vi "Acceleration.vi"() -> ()   [LabVIEW 2020]
uses:
  Control/AccelerationBestRecordIndicator.ctl
  Control/AccelerationCurrentRecordIndicator.ctl
  CommonControl/Flag.ctl
  Control/AccelerationState.ctl
  <vilib>/DAQmx/write.llb/DAQmx Write (Analog 1D DBL NChan 1Samp).vi
  <vilib>/DAQmx/read.llb/DAQmx Read (Analog 1D DBL NChan 1Samp).vi
  <vilib>/DAQmx/create/channels.llb/DAQmx Create Channel (AO-Voltage-Basic).vi
  <vilib>/DAQmx/create/channels.llb/DAQmx Create Channel (AI-Voltage-Basic).vi
  <vilib>/Utility/file.llb/Read Delimited Spreadsheet (string).vi
  <vilib>/DAQmx/miscellaneous.llb/DAQmx Fill In Error Info.vi
  <vilib>/Utility/file.llb/Write Delimited Spreadsheet (string).vi
panel:
  in  "DNF":bool
  out "Event ProgressData":string[][](table)
  in  "DAQDevice":tag
  in  "NextEntry":bool
  in  "Ready":bool
  in  "Retry":bool
  out "CurrentRecordIndicator":T1
  out "BestRecordIndicator":T2
  in  "Stop":bool
  # "2022 KSAE Formula Acceleration Event"
  # "Time :"
  # "Entry :"
  # "#1"
  # "#2"
  # "#3"
  # "#4"
  # "Univ. :"
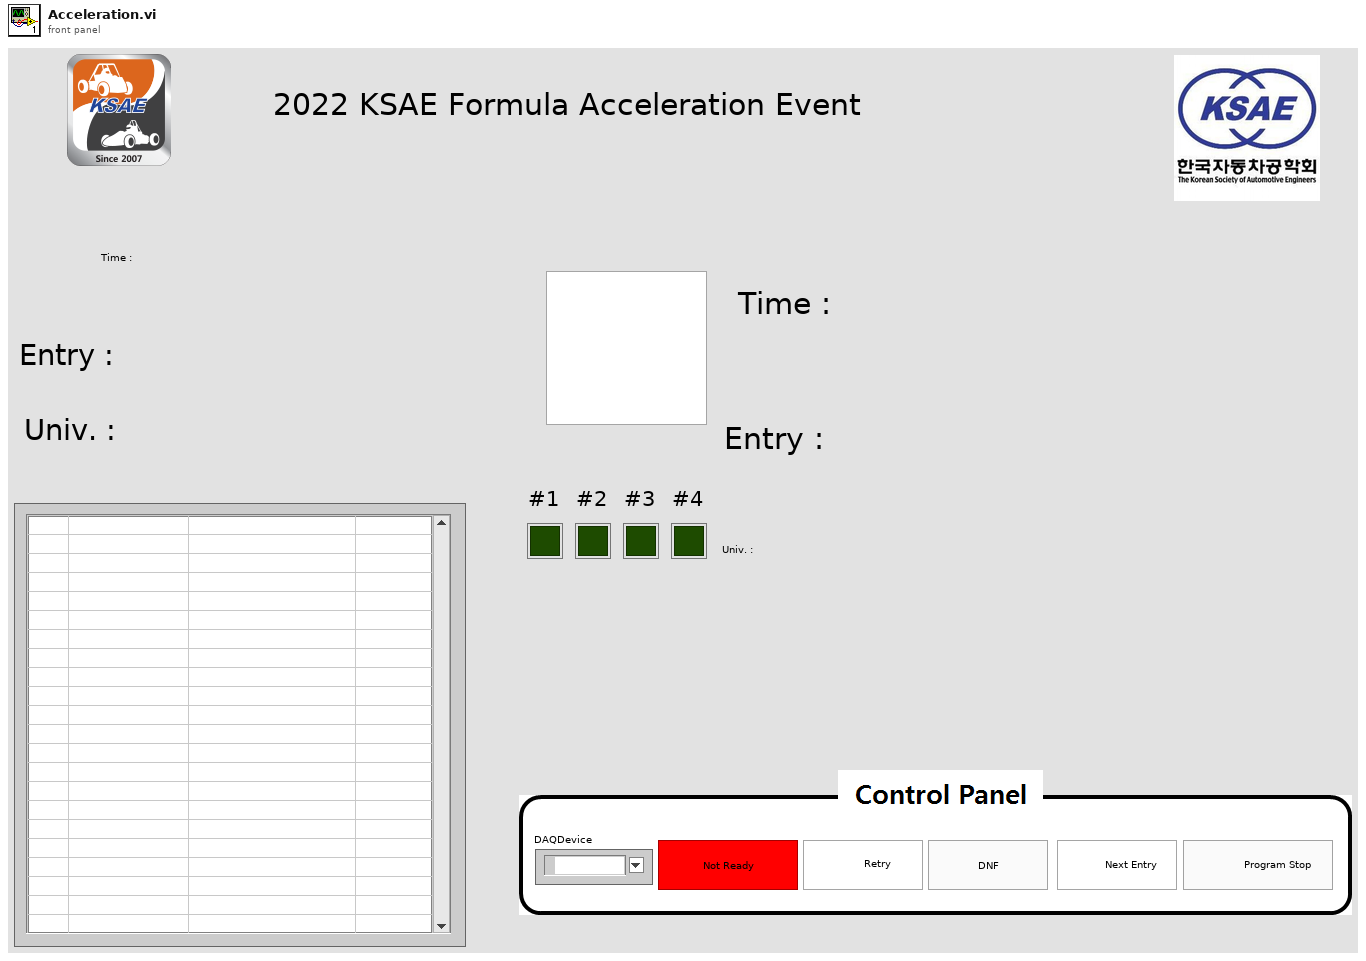
[diagram p1: front panel]
types:
  T1 = typedef "AccelerationCurrentRecordIndicator.ctl" = cluster{"Flag":picture, "Message":string, "Attempt":cluster{"Attempt-1":bool, "Attempt-2":bool, "Attempt-3":bool, "Attempt-4":bool}, "CurrentTime":string, "CurrentEntry":string, "CurrentUniversity":string}
  T2 = typedef "AccelerationBestRecordIndicator.ctl" = cluster{"BestTime":string, "BestEntry":string, "BestUniv":string}
  T3 = typedef "Flag.ctl" = cluster{"GreenFlag":picture, "BlueFlag":picture, "RedFlag":picture, "CheckFlag":picture}
  T4 = typedef "AccelerationState.ctl" = enum16{"Initial", "InputInfomation", "Ready", "Running", "FinshRunning", "LogRecord", "HardwareRelease", "WaittingforNext", "ProgramStop"}
  T5 = cluster{"CurrentRecordIndicator":T1, "BestRecordIndicator":T2, "FlageData":T3, "RefTime(msec)":i64, "Time(msec)":i64, "StateValue":T4, "EventProgress":sgl, "EventProgressData":string[][], "Ready":bool, "Retry":bool, "DNF":bool, "NextEntry":bool, "Stop":bool}
  T6 = cluster{"CurrentEntry":string, "CurrentUniversity":string, "CurrentTeam":string}
  T7 = cluster{"Attempt-1":bool, "Attempt-2":bool, "Attempt-3":bool, "Attempt-4":bool}
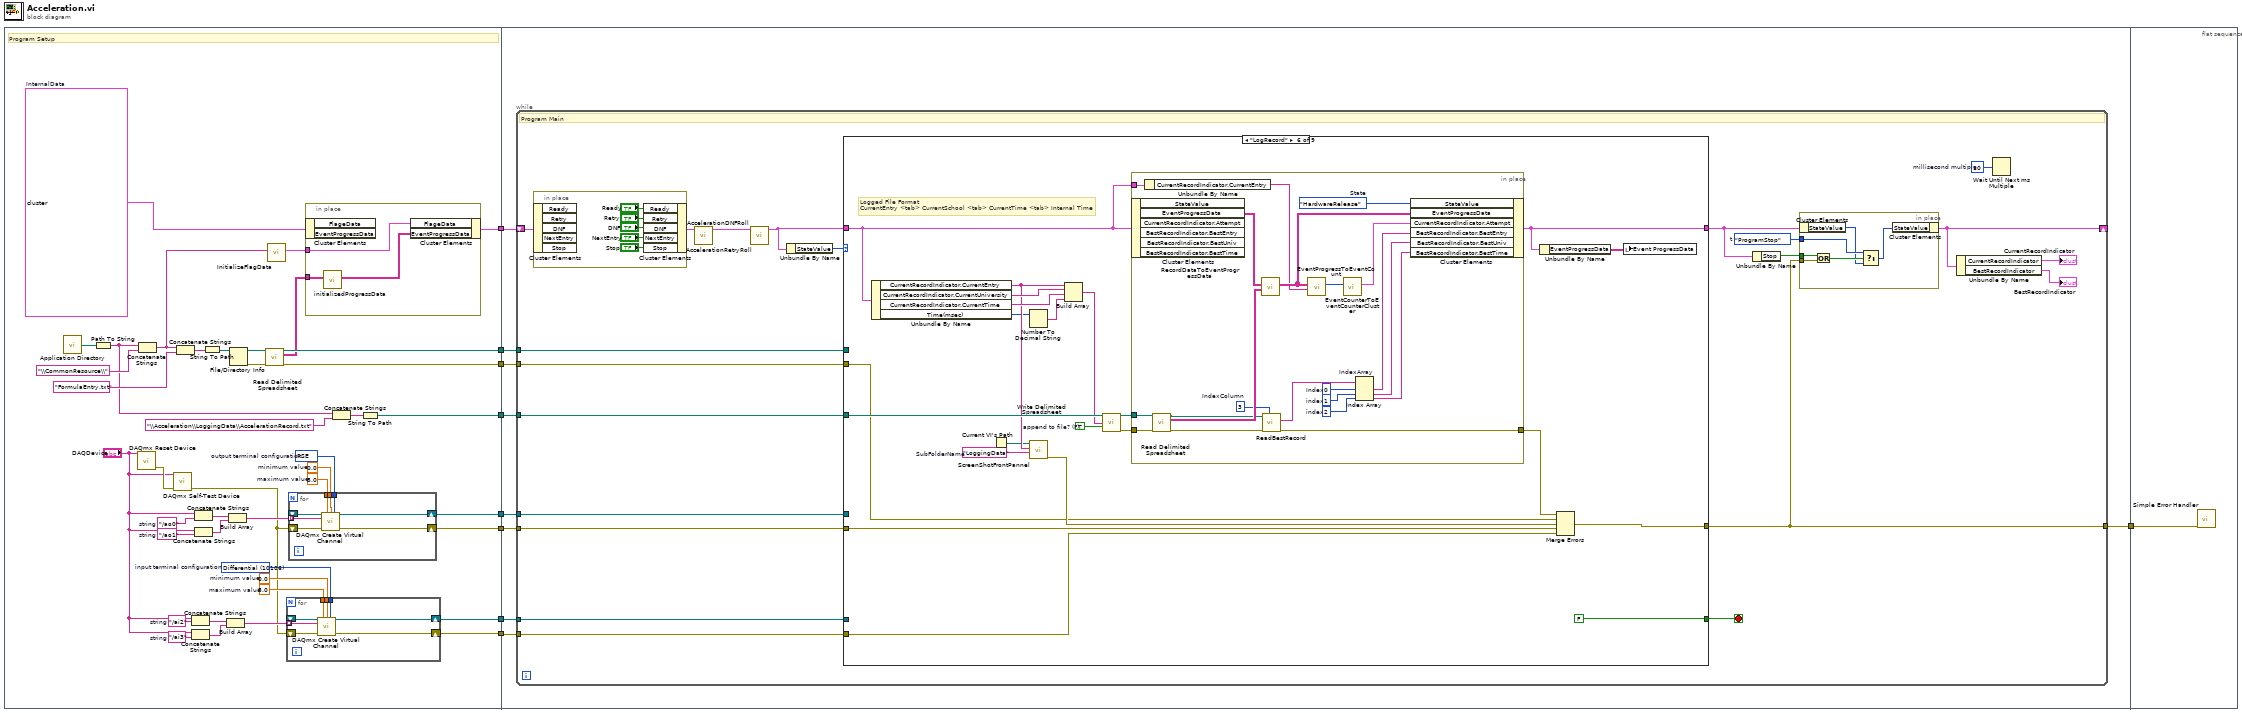
[diagram p0: block diagram]
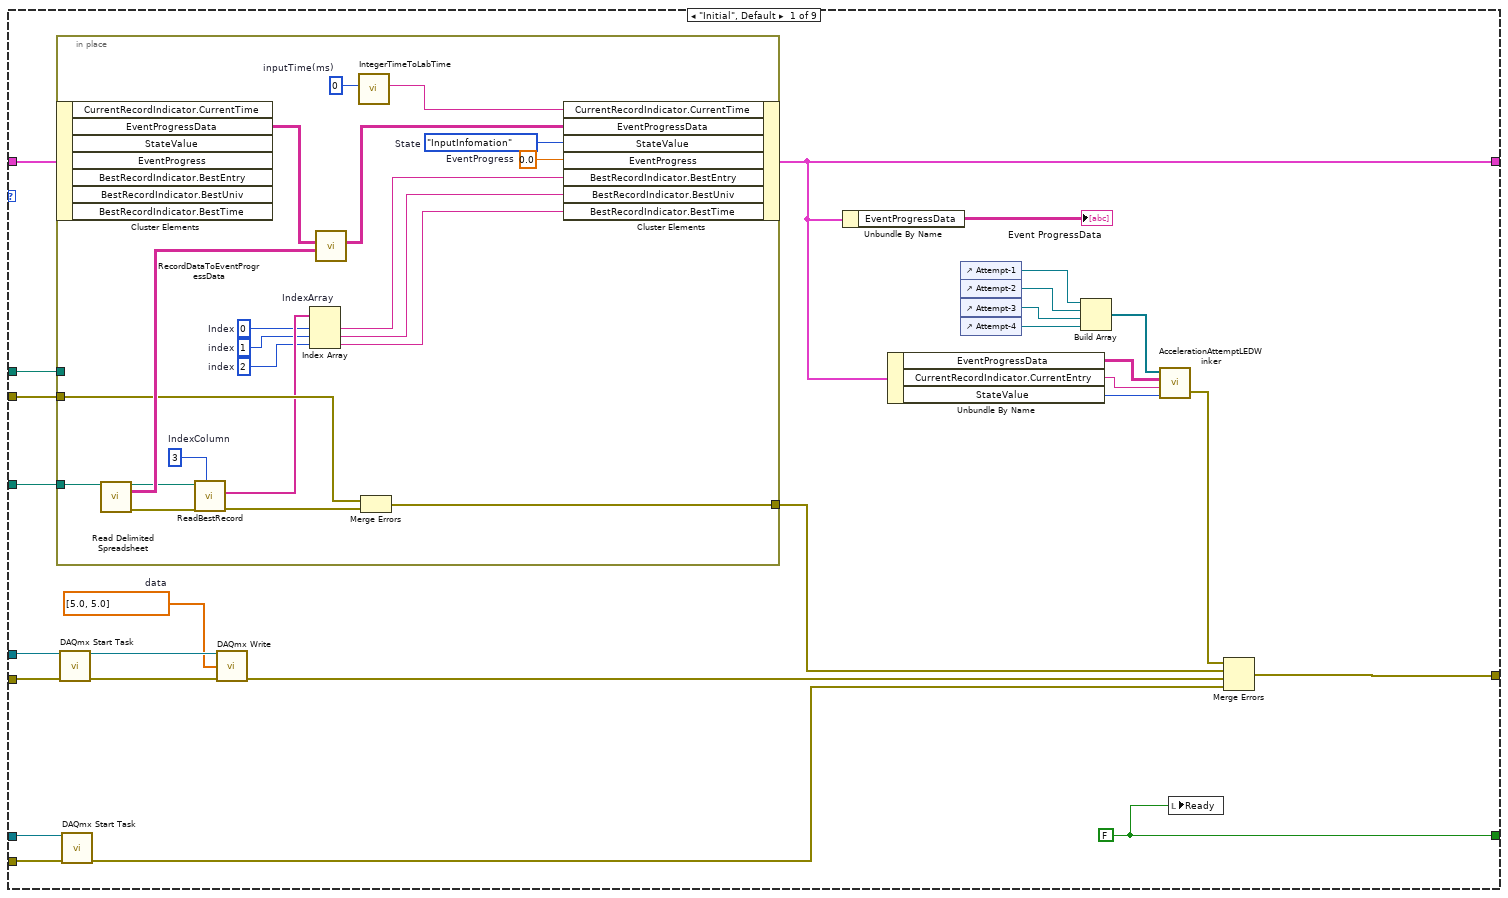
[diagram p2: hidden frame]
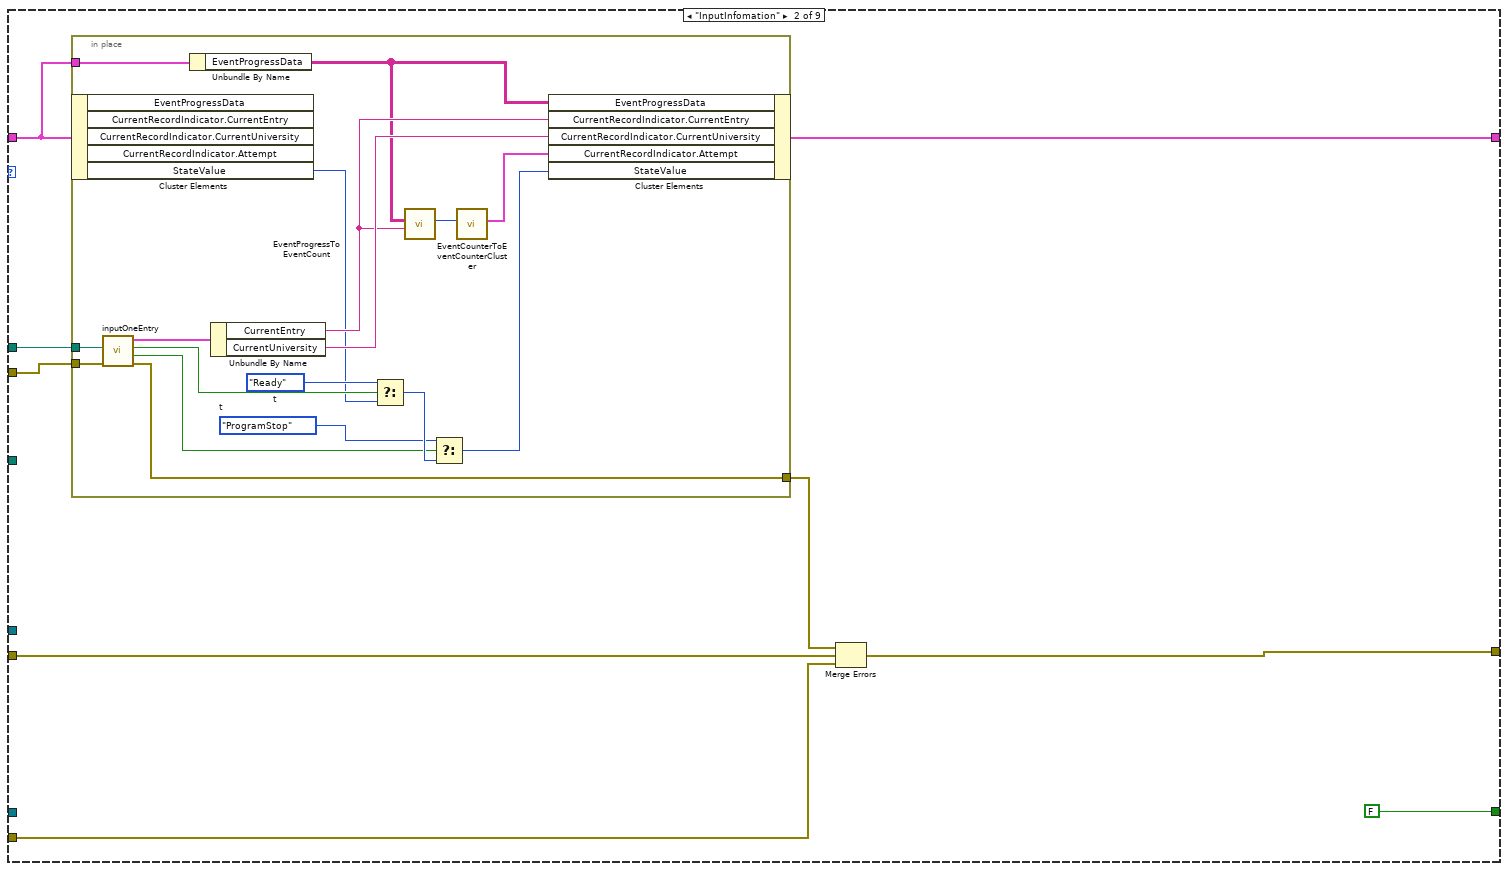
[diagram p3: hidden frame]
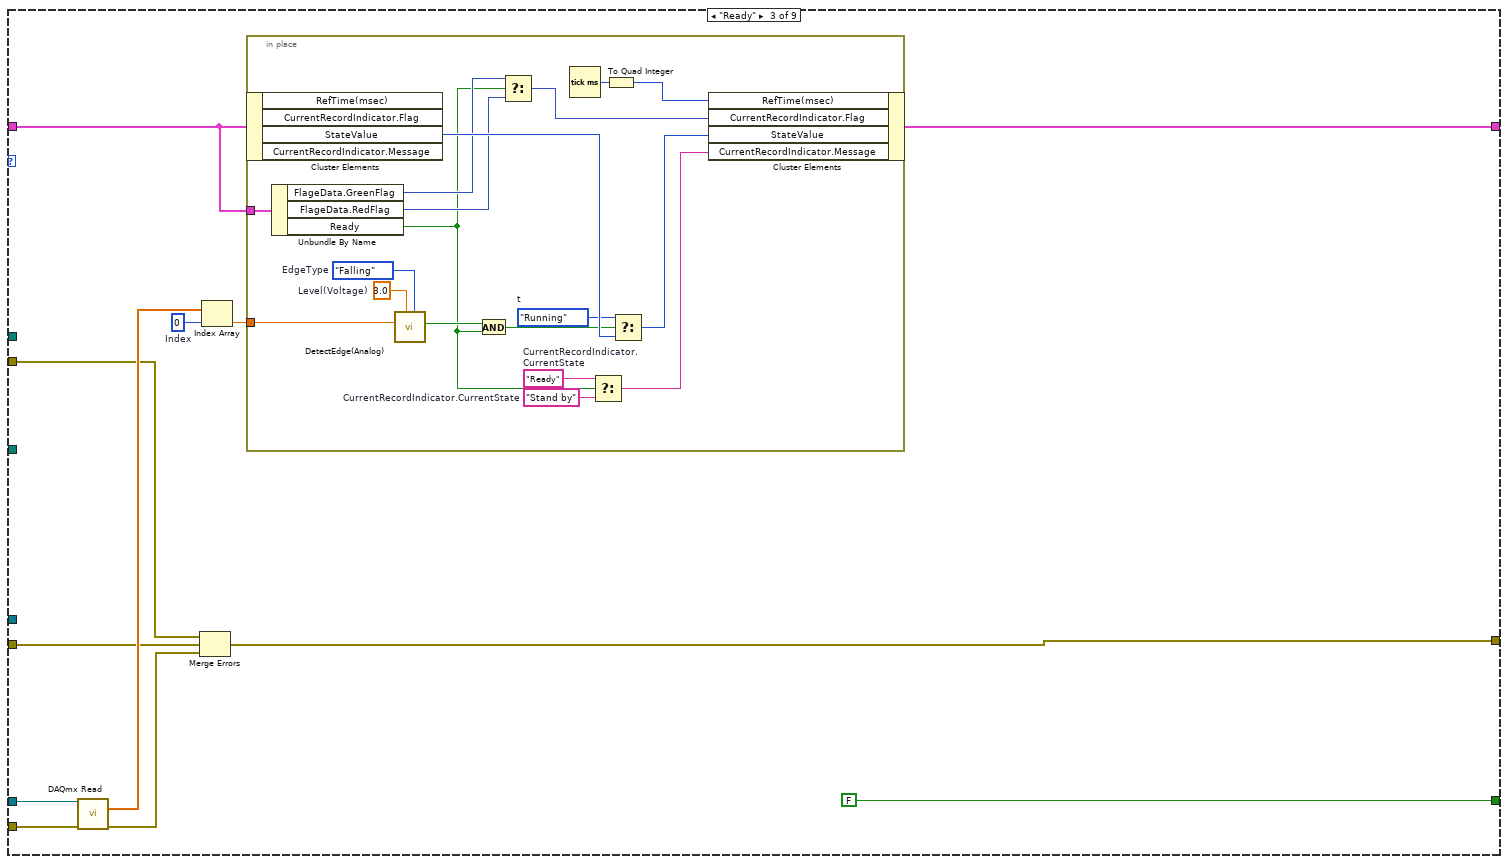
[diagram p4: hidden frame]
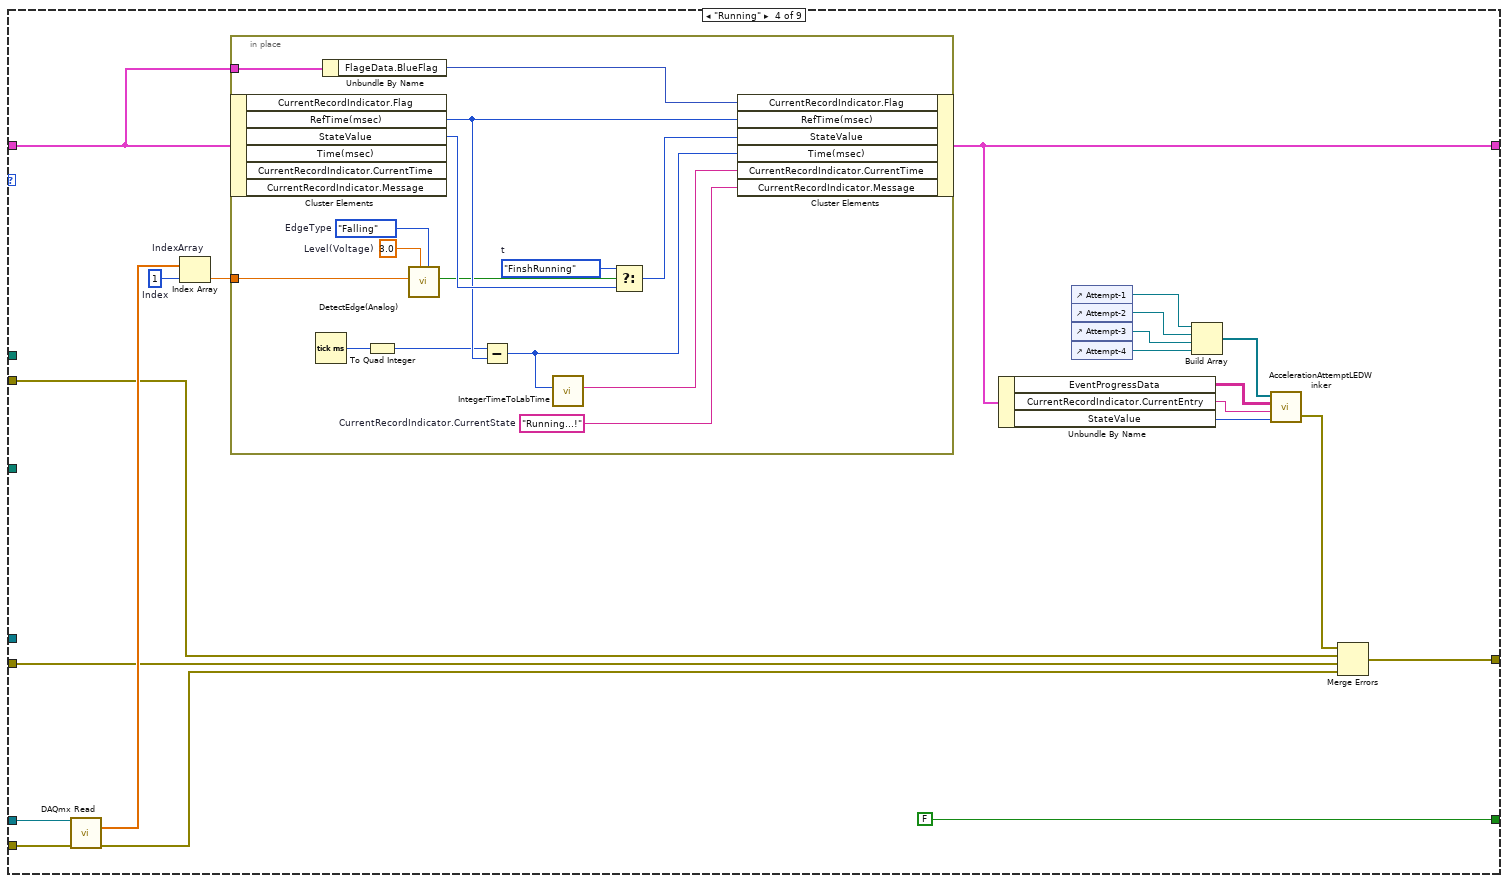
[diagram p5: hidden frame]
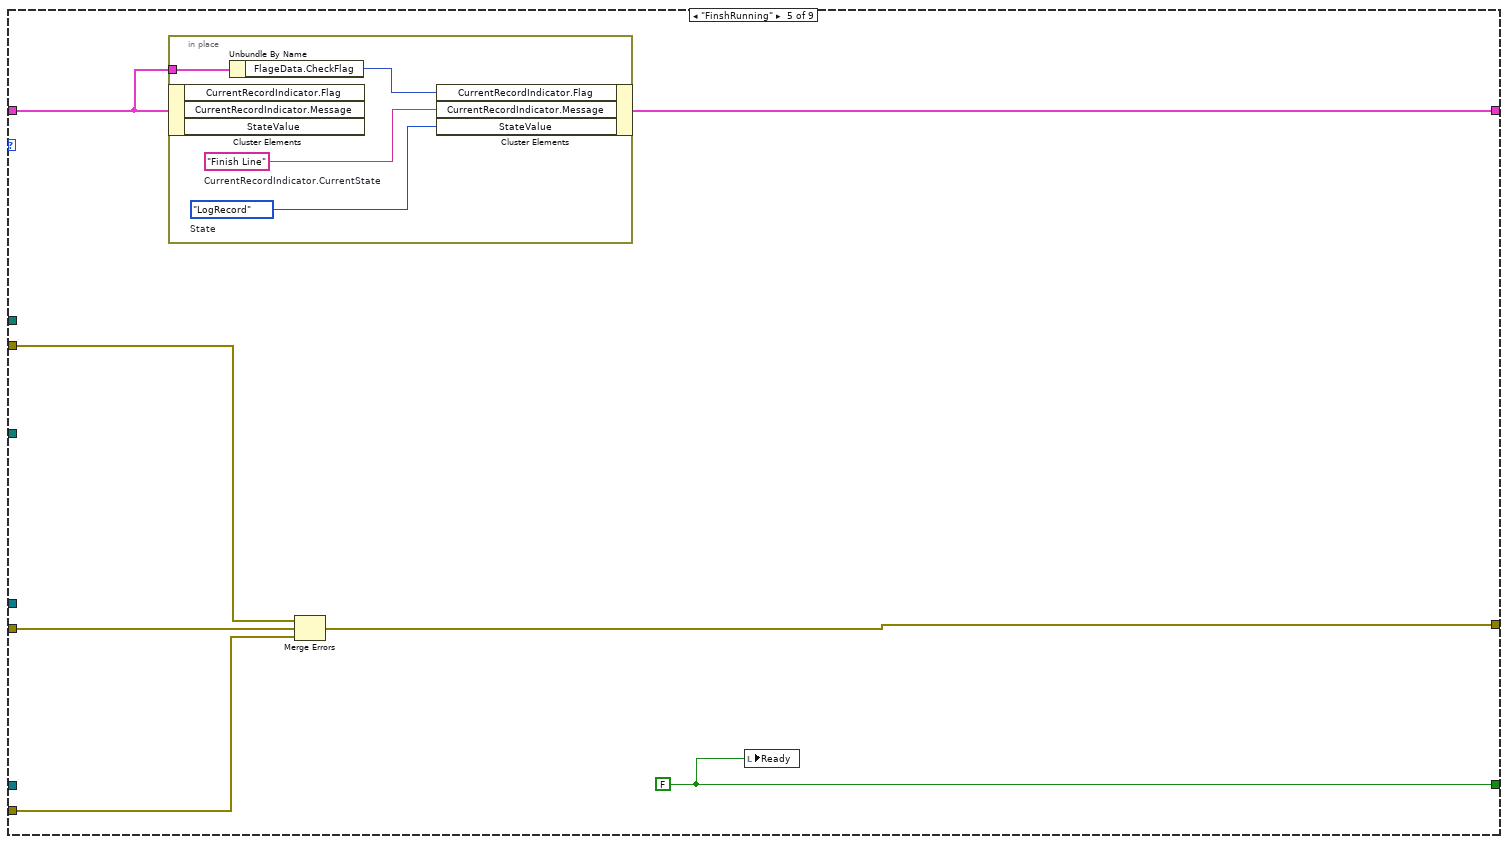
[diagram p6: hidden frame]
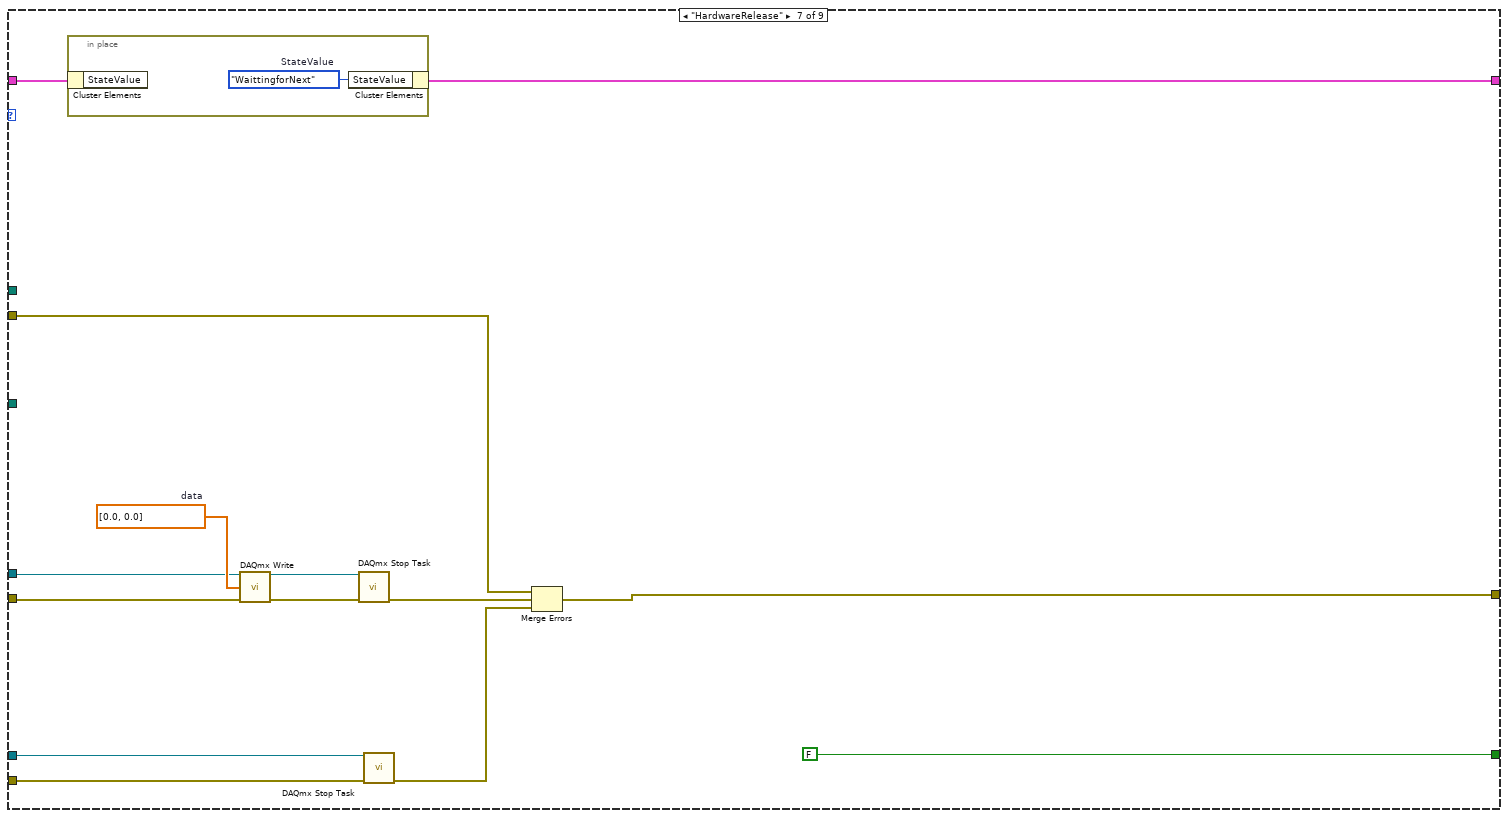
[diagram p7: hidden frame]
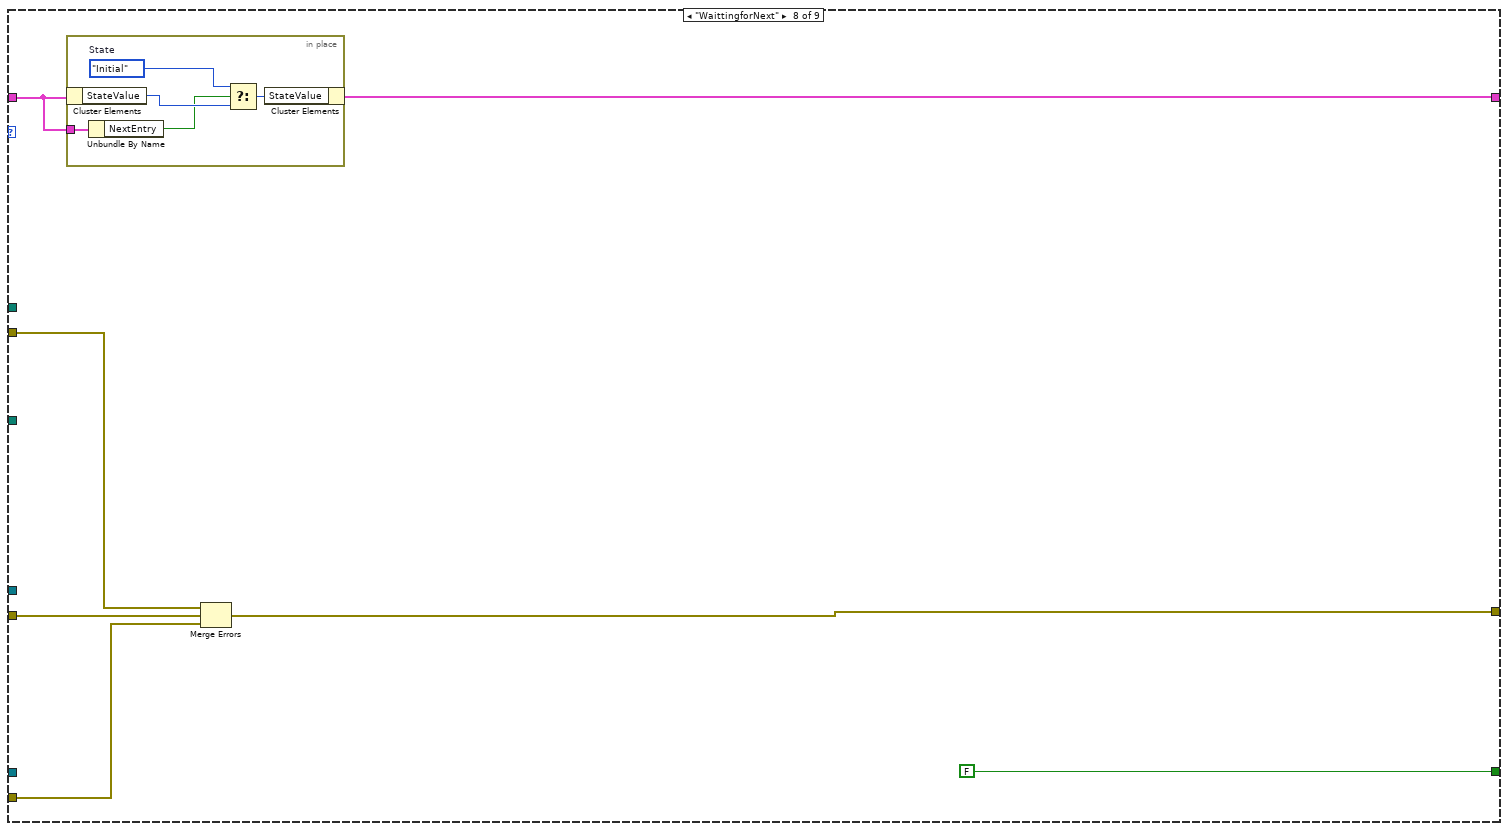
[diagram p8: hidden frame]
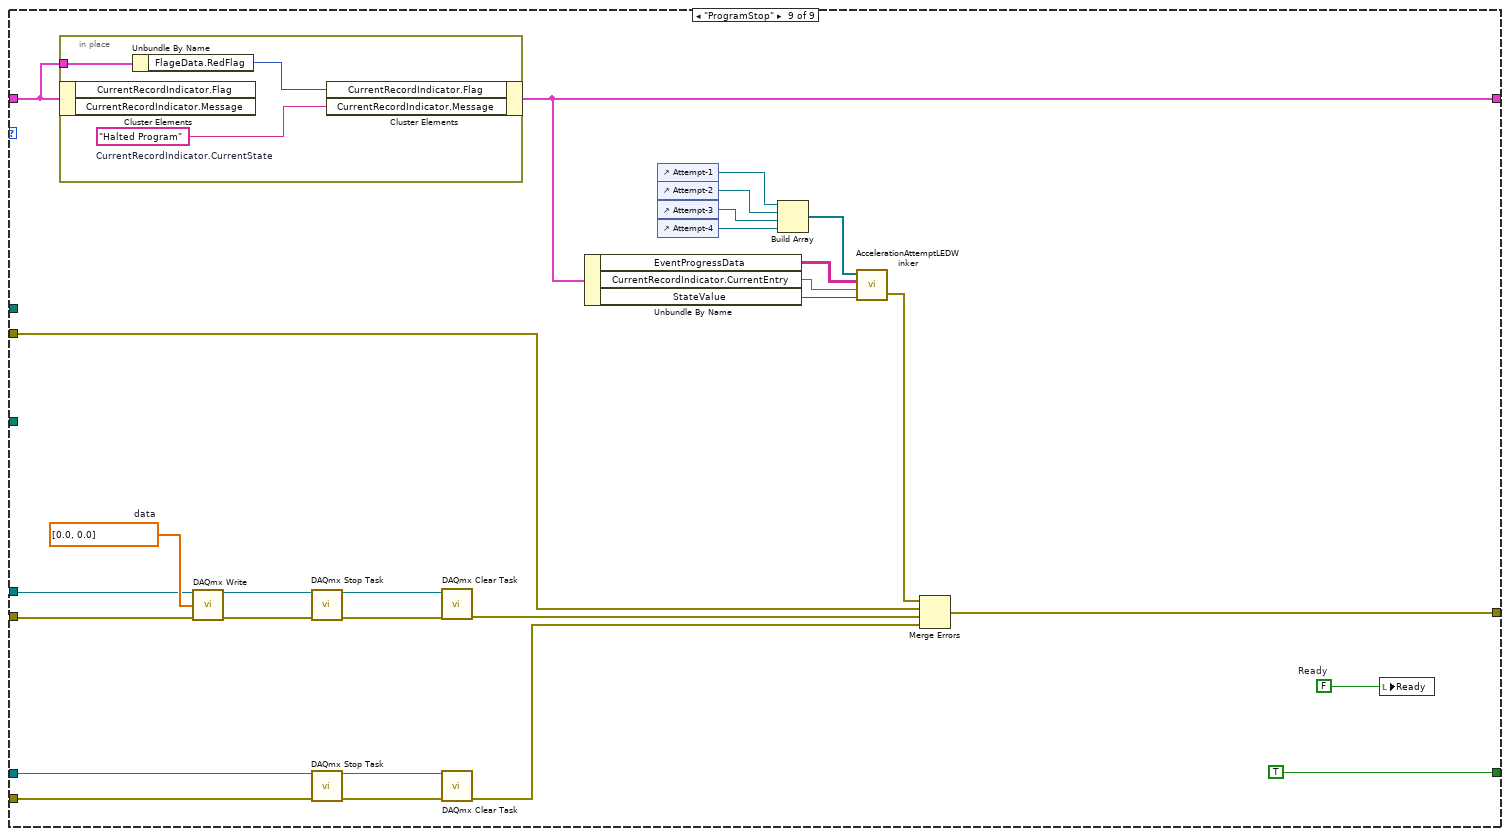
[diagram p9: hidden frame]
diagram:
  n1 = flat-sequence {
    tunnel: [w49] -> w9
    tunnel: [w47] -> w8
    tunnel: [w35] -> w7
    tunnel: [w13] -> w6
    tunnel: [w22] -> w5
    tunnel: [w20] -> w4
    tunnel: [w16] -> w3
    tunnel: [w15] -> w2
    tunnel: w9 -> [w72]
    tunnel: w8 -> [w74]
    tunnel: w7 -> [w75]
    tunnel: w6 -> [w76]
    tunnel: w5 -> [w77]
    tunnel: w4 -> [w69]
    tunnel: w3 -> [w73]
    tunnel: w2 -> [w71]
    tunnel: [w70] -> w1
    tunnel: w1 -> [w362]
    frame #0 {
      w14 = T5 {"CurrentRecordIndicator"={"Flag"=bytes[0], "Message"="", "Attempt"={"Attempt-1"=FALSE, "Attempt-2"=FALSE, "Attempt-3"=FALSE, "Attempt-4"=FALSE}, "CurrentTime"="", "CurrentEntry"="", "CurrentUniversity"=""}, "BestRecordIndicator"={"BestTime"="", "BestEntry"="", "BestUniv"=""}, "FlageData"={"GreenFlag"=bytes[0], "BlueFlag"=bytes[0], "RedFlag"=bytes[0], "CheckFlag"=bytes[0]}, "RefTime(msec)"=0, "Time(msec)"=0, "StateValue"=enum."Initial", "EventProgress"=0.0, "EventProgressData"=[], "Ready"=FALSE, "Retry"=FALSE, "DNF"=FALSE, "NextEntry"=FALSE, "Stop"=FALSE}  # InternalData
      w26 = "/ai3"  # string
      w27 = "/ai2"  # string
      w29 = "/ao1"  # string
      w31 = "/ao0"  # string
      w33 = 5.0  # maximum value
      w32 = 0.0  # minimum value
      w34 = 10106 items=["default"=-1, "RSE"=10083, "NRSE"=10078, "Differential"=10106, "Pseudodifferential"=12529]  # input terminal configuration
      w43 = 10083 items=["Default"=-1, "RSE"=10083, "Differential"=10106, "Pseudodifferential"=12529]  # output terminal configuration
      w44 = 0.0  # minimum value
      w45 = 5.0  # maximum value
      # "Program Setup"
      n2 = call <vilib>:"Application Directory.vi"() -> ("Application Directory"=w42:path)
      n3 = Path To String(path=w42) -> (string=w37:string)
      n4 = call <vilib>:"DAQmx Reset Device.vi"("device in"="DAQDevice") -> ("error out"=w19:errorcluster)  [unwired: 14 in]
      n5 = Concatenate Strings "Concatenate Strings"(w37, "\\CommonResource\\") -> (w11:string)
      n6 = call <vilib>:"DAQmx Self-Test Device.vi"("device in"="DAQDevice", "error in"=w19) -> ("error out"=w17:errorcluster)  [unwired: 13 in]
      n7 = Concatenate Strings(w11, "FormulaEntry.txt") -> (w36:string)
      n8 = Concatenate Strings "Concatenate Strings"("DAQDevice", w27) -> (w25:string)
      n9 = Concatenate Strings "Concatenate Strings"("DAQDevice", w26) -> (w24:string)
      n10 = Concatenate Strings "Concatenate Strings"("DAQDevice", w31) -> (w30:string)
      n11 = Concatenate Strings "Concatenate Strings"("DAQDevice", w29) -> (w28:string)
      n12 = String To Path(string=w36) -> (path=w23:path)
      n13 = Build Array "Build Array"(w25, w24) -> (w48:string[])
      n14 = Build Array "Build Array"(w30, w28) -> (w46:string[])
      n15 = File/Directory Info(path=w23) -> (path out=w22:path, error out=w21:errorcluster)  [unwired: 1 in, 5 out]
      n16 = call-poly <vilib>:"Read Delimited Spreadsheet.vi"("file path (dialog if empty)"=w22, "error in (no error)"=w21) -> ("all rows"=w12:string[][], "error out"=w20:errorcluster)  [unwired: 8 in, 4 out]
      n17 = call "InitializeFlagData.vi"("inputPath"=w11) -> ("outputFlagData"=w10:T3)  [unwired: 9 in, 1 out]
      n18 = for {
        tunnel: w34 -> [w68]
        shift-right: [w67] -> w15
        shift-left: w17 -> [w64]
        shift-right: [w66] -> w49
        shift-left: _ -> [w65]
        tunnel: w33 -> [w63]
        tunnel: w32 -> [w62]
        tunnel: w48 -> [w61] mode=indexing
        n19 = call-poly <vilib>:"DAQmx Create Virtual Channel.vi"("task in"=w65, "maximum value"=w63, "minimum value"=w62, "input terminal configuration"=w68, "physical channels"=w61, "error in"=w64) -> ("task out"=w66:refnum<k21>, "error out"=w67:errorcluster)  [unwired: 8 in]
      }
      n20 = for {
        shift-right: [w60] -> w47
        shift-left: _ -> [w57]
        shift-right: [w59] -> w16
        shift-left: w17 -> [w56]
        tunnel: w46 -> [w58] mode=indexing
        tunnel: w45 -> [w55]
        tunnel: w44 -> [w54]
        tunnel: w43 -> [w53]
        n21 = call-poly <vilib>:"DAQmx Create Virtual Channel.vi"("task in"=w57, "maximum value"=w55, "minimum value"=w54, "output terminal configuration"=w53, "physical channels"=w58, "error in"=w56) -> ("task out"=w60:refnum<k21>, "error out"=w59:errorcluster)  [unwired: 8 in]
      }
      n22 = in-place {
        in-place-border: w10 -> [w50]
        in-place-border: w12 -> [w52]
        n23 = in-place-cluster #1(w14) -> ()  [unwired: 2 out]
        n24 = call "initializedProgressData.vi"("inputEntry"=w52) -> ("outputProgressData"=w51:string[][])  [unwired: 10 in]
        n25 = in-place-cluster #1("FlageData"=w50, "EventProgressData"=w51) -> (w13:T5)
      }
      n26 = Concatenate Strings "Concatenate Strings"(w37, "\\Acceleration\\LoggingData\\AccelerationRecord.txt") -> (w40:string)
      n27 = String To Path(string=w40) -> (path=w35:path)
    }
    frame #1 {
      n28 = while {
        tunnel: w72 -> [w98]
        shift-right: [w84] -> _
        shift-left: w76 -> [w88]
        tunnel: w74 -> [w94]
        tunnel: w75 -> [w93]
        tunnel: w77 -> [w91]
        tunnel: w73 -> [w90]
        tunnel: w71 -> [w89]
        tunnel: [w78] -> w70
        tunnel: w69 -> [w87]
        stop <- w95 stop-if-true
        w85 = AccelerationState."ProgramStop"  # t
        w92 = u32 10  # millisecond multiple
        # "Program Main"
        n29 = in-place {
          n30 = in-place-cluster #2(w88) -> ()  [unwired: 5 out]
          n31 = in-place-cluster #2("Ready"="Ready", "Retry"="Retry", "DNF"="DNF", "NextEntry"="NextEntry", "Stop"="Stop") -> (w82:T5)
        }
        n32 = call "AccelerationDNFRoll.vi"("inputInternalData"=w82) -> ("outputInternalData"=w81:T5)  [unwired: 10 in]
        n33 = call "AccelerationRetryRoll.vi"("inputInternalData"=w81) -> ("outputInternalData"=w80:T5)  [unwired: 10 in]
        n34 = Unbundle By Name(w80) -> ("StateValue"=w79:T4)
        n35 = case shown="\"LogRecord\"" w79 {
          tunnel: w98 -> [w124 _ w189 w228 _ _ w306 _ w352]
          tunnel: w89 -> [w123 w153 w188 w227 w249 w266 w305 w316 w338]
          tunnel: w80 -> [w130 w152 w181 w221 w248 w257 w300 w313 w336]
          tunnel: [w106 w157 w187 w210 w250 w265 w299 w318 w327] -> w83
          tunnel: [w105 FALSE FALSE FALSE w244 FALSE FALSE FALSE TRUE] -> w95
          tunnel: [w120 w159 w180 w220 w247 w272 w302 w317 w348] -> w78
          tunnel: w94 -> [w126 _ _ _ _ _ w308 _ w343]
          tunnel: w93 -> [w116 _ _ _ _ w273 _ _ _]
          tunnel: w91 -> [w119 w156 _ _ _ _ _ _ _]
          tunnel: w90 -> [w125 w154 w179 w219 w246 w267 w307 w315 w342]
          tunnel: w87 -> [w118 w155 w178 w218 w245 w256 w298 w314 w326]
          frame "Initial", Default {
            w127 = dbl[] [5.0, 5.0]  # data
            w105 = FALSE
            n36 = in-place {
              in-place-border: w119 -> [_]
              in-place-border: w118 -> [w142]
              in-place-border: [w143] -> w117
              in-place-border: w116 -> [w144]
              w137 = 2  # index
              w138 = 1  # index
              w139 = 3  # IndexColumn
              w140 = 0  # Index
              w149 = i64 0  # inputTime(ms)
              w150 = sgl 0.0  # EventProgress
              w151 = AccelerationState."InputInfomation"  # State
              n37 = in-place-cluster #3(w130) -> ("EventProgressData"=w146:string[][])  [unwired: 6 out]
              n38 = call-poly <vilib>:"Read Delimited Spreadsheet.vi"("file path (dialog if empty)"=w144) -> ("new file path (Not A Path if cancelled)"=w136:path, "all rows"=w147:string[][], "error out"=w135:errorcluster)  [unwired: 9 in, 3 out]
              n39 = call "ReadBestRecord.vi"("IndexColumn"=w139, "ErrorInput"=w135, "FilepathInput"=w136) -> ("ErrorOutput"=w134:errorcluster, "Data"=w141:string[])  [unwired: 6 in, 1 out]
              n40 = Index Array "IndexArray"(array=w141, index #1=w140, index #2=w138, index #3=w137) -> (element #1=w133:string, element #2=w132:string, element #3=w131:string)
              n41 = call "RecordDataToEventProgressData.vi"("RecordData"=w147, "inputEventProgressData"=w146) -> ("outputEventProgressData"=w145:string[][])  [unwired: 9 in]
              n42 = call "IntegerTimeToLabTime.vi"("inputTime(msec)"=w149) -> ("outputTime(mm-ss-sss)"=w148:string)  [unwired: 10 in]
              n43 = Merge Errors "Merge Errors"(w142, w134) -> (w143:errorcluster)
              n44 = in-place-cluster #3("CurrentRecordIndicator.CurrentTime"=w148, "EventProgressData"=w145, "StateValue"=w151, "EventProgress"=w150, "BestRecordIndicator.BestEntry"=w133, "BestRecordIndicator.BestUniv"=w132, "BestRecordIndicator.BestTime"=w131) -> (w106:T5)
            }
            n45 = call <vilib>:"DAQmx Start Task.vi"("task/channels in"=w126, "error in"=w125) -> ("task out"=w129:refnum<k21>, "error out"=w128:errorcluster)  [unwired: 12 in]
            n46 = call <vilib>:"DAQmx Start Task.vi"("task/channels in"=w124, "error in"=w123) -> ("error out"=w121:errorcluster)  [unwired: 12 in, 1 out]
            n47 = call-poly <vilib>:"DAQmx Write.vi"("task/channels in"=w129, "data"=w127, "error in"=w128) -> ("error out"=w122:errorcluster)  [unwired: 10 in, 2 out]
            n48 = Unbundle By Name(w106) -> ("EventProgressData"=→"Event ProgressData":string[][])
            n49 = Unbundle By Name(w106) -> ("EventProgressData"=w113:string[][], "CurrentRecordIndicator.CurrentEntry"=w114:string, "StateValue"=w107:T4)
            n50 = control-ref of="Attempt-1"() -> (w111:refnum<vi>)
            n51 = control-ref of="Attempt-2"() -> (w110:refnum<vi>)
            n52 = control-ref of="Attempt-3"() -> (w109:refnum<vi>)
            n53 = control-ref of="Attempt-4"() -> (w108:refnum<vi>)
            n54 = Build Array(w111, w110, w109, w108) -> (w112:refnum<vi>[])
            n55 = call "AccelerationAttemptLEDWinker.vi"("StateValue"=w107, "CurrentEntry"=w114, "EventProgressDataInput"=w113, "inputRefOfLED"=w112) -> ("outputError"=w104:errorcluster)  [unwired: 7 in]
            n56 = local write "Ready"(w105) -> ()
            n57 = Merge Errors "Merge Errors"(w104, w117, w122, w121) -> (w120:errorcluster)
          }
          frame "InputInfomation" {
            n58 = in-place {
              in-place-border: [w174] -> w158
              in-place-border: w156 -> [w167]
              in-place-border: w152 -> [w171]
              in-place-border: w155 -> [w168]
              w175 = AccelerationState."ProgramStop"  # t
              w177 = AccelerationState."Ready"  # t
              n59 = in-place-cluster #4(w152) -> ("StateValue"=w162:T4)  [unwired: 4 out]
              n60 = call "inputOneEntry.vi"("inputError"=w168, "file path (dialog if empty)"=w167) -> ("outputError"=w174:errorcluster, "StopButtonOutput"=w164:bool, "OKButtonOutput"=w165:bool, "CurrentData"=w166:T6)  [unwired: 6 in]
              n61 = Unbundle By Name(w171) -> ("EventProgressData"=w163:string[][])
              n62 = Unbundle By Name(w166) -> ("CurrentEntry"=w172:string, "CurrentUniversity"=w173:string)
              n63 = Select(t=w177, s=w165, f=w162) -> (s? t:f=w176:T4)
              n64 = call "EventProgressToEventCount.vi"("CurrentEntry"=w172, "EventProgressDataInput"=w163) -> ("EventCount"=w170:i32)  [unwired: 9 in]
              n65 = Select(t=w175, s=w164, f=w176) -> (s? t:f=w161:T4)
              n66 = call "EventCounterToEventCounterCluster.vi"("EventCount"=w170) -> ("CurrentRecordIndicator.EventCount"=w169:T7)  [unwired: 10 in]
              n67 = in-place-cluster #4("EventProgressData"=w163, "CurrentRecordIndicator.CurrentEntry"=w172, "CurrentRecordIndicator.CurrentUniversity"=w173, "CurrentRecordIndicator.Attempt"=w169, "StateValue"=w161) -> (w157:T5)
            }
            n68 = Merge Errors "Merge Errors"(w158, w154, w153) -> (w159:errorcluster)
          }
          frame "Ready" {
            w185 = 0  # Index
            n69 = call-poly <vilib>:"DAQmx Read.vi"("task/channels in"=w189, "error in"=w188) -> ("data"=w184:dbl[], "error out"=w186:errorcluster)  [unwired: 11 in, 1 out]
            n70 = Merge Errors "Merge Errors"(w178, w179, w186) -> (w180:errorcluster)
            n71 = Index Array "Index Array"(array=w184, index=w185) -> (element=w183:dbl)
            n72 = in-place {
              in-place-border: w183 -> [w190]
              in-place-border: w181 -> [w197]
              w193 = enum16{"Rising", "Falling"}."Falling"  # EdgeType
              w198 = "Stand by"  # CurrentRecordIndicator.CurrentState
              w201 = 3.0  # Level(Voltage)
              w199 = "Ready"  # CurrentRecordIndicator.CurrentState
              w206 = AccelerationState."Running"  # t
              n73 = in-place-cluster #5(w181) -> ("StateValue"=w207:T4)  [unwired: 3 out]
              n74 = Unbundle By Name(w197) -> ("FlageData.GreenFlag"=w195:picture, "FlageData.RedFlag"=w196:picture, "Ready"=w192:bool)
              n75 = call "DetectEdge(Analog).vi"("EdgeType"=w193, "Level(Voltage)"=w201, "Voltage"=w190) -> ("DetectedEdge"=w205:bool)  [unwired: 8 in]
              n76 = And(x=w205, y=w192) -> (x .and. y?=w203:bool)
              n77 = Select(t=w195, s=w192, f=w196) -> (s? t:f=w202:picture)
              n78 = Tick Count (ms)() -> (millisecond timer value=w204:u32)
              n79 = Select(t=w199, s=w192, f=w198) -> (s? t:f=w200:string)
              n80 = To Quad Integer(1:w204) -> (0:w194:i64)
              n81 = Select(t=w206, s=w203, f=w207) -> (s? t:f=w191:T4)
              n82 = in-place-cluster #5("RefTime(msec)"=w194, "CurrentRecordIndicator.Flag"=w202, "StateValue"=w191, "CurrentRecordIndicator.Message"=w200) -> (w187:T5)
            }
          }
          frame "Running" {
            w223 = 1  # Index
            n83 = call-poly <vilib>:"DAQmx Read.vi"("task/channels in"=w228, "error in"=w227) -> ("data"=w226:dbl[], "error out"=w224:errorcluster)  [unwired: 11 in, 1 out]
            n84 = Index Array "IndexArray"(array=w226, index=w223) -> (element=w222:dbl)
            n85 = in-place {
              in-place-border: w222 -> [w229]
              in-place-border: w221 -> [w234]
              w232 = enum16{"Rising", "Falling"}."Falling"  # EdgeType
              w236 = 3.0  # Level(Voltage)
              w239 = "Running...!"  # CurrentRecordIndicator.CurrentState
              w242 = AccelerationState."FinshRunning"  # t
              n86 = in-place-cluster #6(w221) -> ("RefTime(msec)"=w238:i64, "StateValue"=w243:T4)  [unwired: 4 out]
              n87 = Tick Count (ms)() -> (millisecond timer value=w241:u32)
              n88 = Unbundle By Name(w234) -> ("FlageData.BlueFlag"=w233:picture)
              n89 = To Quad Integer(1:w241) -> (0:w235:i64)
              n90 = call "DetectEdge(Analog).vi"("EdgeType"=w232, "Level(Voltage)"=w236, "Voltage"=w229) -> ("DetectedEdge"=w237:bool)  [unwired: 8 in]
              n91 = Subtract(x=w235, y=w238) -> (x-y=w230:i64)
              n92 = call "IntegerTimeToLabTime.vi"("inputTime(msec)"=w230) -> ("outputTime(mm-ss-sss)"=w240:string)  [unwired: 10 in]
              n93 = Select(t=w242, s=w237, f=w243) -> (s? t:f=w231:T4)
              n94 = in-place-cluster #6("CurrentRecordIndicator.Flag"=w233, "RefTime(msec)"=w238, "StateValue"=w231, "Time(msec)"=w230, "CurrentRecordIndicator.CurrentTime"=w240, "CurrentRecordIndicator.Message"=w239) -> (w210:T5)
            }
            n95 = Unbundle By Name(w210) -> ("EventProgressData"=w216:string[][], "CurrentRecordIndicator.CurrentEntry"=w217:string, "StateValue"=w209:T4)
            n96 = control-ref of="Attempt-1"() -> (w214:refnum<vi>)
            n97 = control-ref of="Attempt-2"() -> (w213:refnum<vi>)
            n98 = control-ref of="Attempt-3"() -> (w212:refnum<vi>)
            n99 = control-ref of="Attempt-4"() -> (w211:refnum<vi>)
            n100 = Build Array(w214, w213, w212, w211) -> (w215:refnum<vi>[])
            n101 = call "AccelerationAttemptLEDWinker.vi"("StateValue"=w209, "CurrentEntry"=w217, "EventProgressDataInput"=w216, "inputRefOfLED"=w215) -> ("outputError"=w208:errorcluster)  [unwired: 7 in]
            n102 = Merge Errors "Merge Errors"(w208, w218, w219, w224) -> (w220:errorcluster)
          }
          frame "FinshRunning" {
            w244 = FALSE
            n103 = in-place {
              in-place-border: w248 -> [w252]
              w253 = AccelerationState."LogRecord"  # State
              w254 = "Finish Line"  # CurrentRecordIndicator.CurrentState
              n104 = in-place-cluster #7(w248) -> ()  [unwired: 3 out]
              n105 = Unbundle By Name(w252) -> ("FlageData.CheckFlag"=w251:picture)
              n106 = in-place-cluster #7("CurrentRecordIndicator.Flag"=w251, "CurrentRecordIndicator.Message"=w254, "StateValue"=w253) -> (w250:T5)
            }
            n107 = Merge Errors "Merge Errors"(w245, w246, w249) -> (w247:errorcluster)
            n108 = local write "Ready"(w244) -> ()
          }
          frame "LogRecord" {
            w259 = TRUE  # append to file? (F)
            w268 = "LoggingData"  # SubFolderName
            # "Logged File Format\nCurrentEntry <tab> CurrentSchool <tab> CurrentTime <tab> Internal Time"
            n109 = Unbundle By Name(w257) -> ("CurrentRecordIndicator.CurrentEntry"=w270:string, "CurrentRecordIndicator.CurrentUniversity"=w276:string, "CurrentRecordIndicator.CurrentTime"=w275:string, "Time(msec)"=w258:i64)
            n110 = Current VI's Path() -> (path=w269:path)
            n111 = Number To Decimal String(number=w258) -> (decimal integer string=w274:string)  [unwired: 1 in]
            n112 = call "ScreenShotFrontPannel.vi"("SubFolderName"=w268, "FileName"=w270, "vi path"=w269) -> ("error out"=w271:errorcluster)  [unwired: 8 in]
            n113 = Build Array "Build Array"(w270, w276, w275, w274) -> (w260:string[])
            n114 = call-poly <vilib>:"Write Delimited Spreadsheet.vi"("file path (dialog if empty)"=w273, "1D data"=w260, "append to file? (new file:F)"=w259) -> ("new file path (Not A Path if cancelled)"=w262:path, "error out"=w263:errorcluster)  [unwired: 11 in]
            n115 = in-place {
              in-place-border: w263 -> [w297]
              in-place-border: w262 -> [w296]
              in-place-border: [w277] -> w261
              in-place-border: w257 -> [w292]
              w283 = 2  # index
              w284 = 1  # index
              w285 = 3  # IndexColumn
              w286 = 0  # Index
              w293 = AccelerationState."HardwareRelease"  # State
              n116 = in-place-cluster #8(w257) -> ("EventProgressData"=w295:string[][])  [unwired: 5 out]
              n117 = Unbundle By Name(w292) -> ("CurrentRecordIndicator.CurrentEntry"=w290:string)
              n118 = call-poly <vilib>:"Read Delimited Spreadsheet.vi"("file path (dialog if empty)"=w296, "error in (no error)"=w297) -> ("new file path (Not A Path if cancelled)"=w281:path, "all rows"=w294:string[][], "error out"=w282:errorcluster)  [unwired: 8 in, 3 out]
              n119 = call "RecordDataToEventProgressData.vi"("RecordData"=w294, "inputEventProgressData"=w295) -> ("outputEventProgressData"=w291:string[][])  [unwired: 9 in]
              n120 = call "ReadBestRecord.vi"("IndexColumn"=w285, "ErrorInput"=w282, "FilepathInput"=w281) -> ("ErrorOutput"=w277:errorcluster, "Data"=w287:string[])  [unwired: 6 in, 1 out]
              n121 = call "EventProgressToEventCount.vi"("CurrentEntry"=w290, "EventProgressDataInput"=w291) -> ("EventCount"=w289:i32)  [unwired: 9 in]
              n122 = call "EventCounterToEventCounterCluster.vi"("EventCount"=w289) -> ("CurrentRecordIndicator.EventCount"=w288:T7)  [unwired: 10 in]
              n123 = Index Array "IndexArray"(array=w287, index #1=w286, index #2=w284, index #3=w283) -> (element #1=w280:string, element #2=w279:string, element #3=w278:string)
              n124 = in-place-cluster #8("StateValue"=w293, "EventProgressData"=w291, "CurrentRecordIndicator.Attempt"=w288, "BestRecordIndicator.BestEntry"=w280, "BestRecordIndicator.BestUniv"=w279, "BestRecordIndicator.BestTime"=w278) -> (w265:T5)
            }
            n125 = Unbundle By Name(w265) -> ("EventProgressData"=w264:string[][])
            n126 = Merge Errors "Merge Errors"(w261, w256, w271, w267, w266) -> (w272:errorcluster)
            n127 = local write "Event ProgressData"(w264) -> ()
          }
          frame "HardwareRelease" {
            w311 = dbl[] [0.0, 0.0]  # data
            n128 = in-place {
              w312 = AccelerationState."WaittingforNext"  # StateValue
              n129 = in-place-cluster #9(w300) -> ()  [unwired: 1 out]
              n130 = in-place-cluster #9("StateValue"=w312) -> (w299:T5)
            }
            n131 = call-poly <vilib>:"DAQmx Write.vi"("task/channels in"=w308, "data"=w311, "error in"=w307) -> ("task out"=w310:refnum<k21>, "error out"=w309:errorcluster)  [unwired: 10 in, 1 out]
            n132 = call <vilib>:"DAQmx Stop Task.vi"("task/channels in"=w310, "error in"=w309) -> ("error out"=w304:errorcluster)  [unwired: 12 in, 1 out]
            n133 = call <vilib>:"DAQmx Stop Task.vi"("task/channels in"=w306, "error in"=w305) -> ("error out"=w303:errorcluster)  [unwired: 12 in, 1 out]
            n134 = Merge Errors "Merge Errors"(w298, w304, w303) -> (w302:errorcluster)
          }
          frame "WaittingforNext" {
            n135 = in-place {
              in-place-border: w313 -> [w321]
              w324 = AccelerationState."Initial"  # State
              n136 = in-place-cluster #10(w313) -> ("StateValue"=w323:T4)
              n137 = Unbundle By Name(w321) -> ("NextEntry"=w320:bool)
              n138 = Select(t=w324, s=w320, f=w323) -> (s? t:f=w322:T4)
              n139 = in-place-cluster #10("StateValue"=w322) -> (w318:T5)
            }
            n140 = Merge Errors "Merge Errors"(w314, w315, w316) -> (w317:errorcluster)
          }
          frame "ProgramStop" {
            w346 = dbl[] [0.0, 0.0]  # data
            w350 = FALSE  # Ready
            n141 = in-place {
              in-place-border: w336 -> [w354]
              w355 = "Halted Program"  # CurrentRecordIndicator.CurrentState
              n142 = in-place-cluster #11(w336) -> ()  [unwired: 2 out]
              n143 = Unbundle By Name(w354) -> ("FlageData.RedFlag"=w353:picture)
              n144 = in-place-cluster #11("CurrentRecordIndicator.Flag"=w353, "CurrentRecordIndicator.Message"=w355) -> (w327:T5)
            }
            n145 = call-poly <vilib>:"DAQmx Write.vi"("task/channels in"=w343, "data"=w346, "error in"=w342) -> ("task out"=w345:refnum<k21>, "error out"=w344:errorcluster)  [unwired: 10 in, 1 out]
            n146 = call <vilib>:"DAQmx Stop Task.vi"("task/channels in"=w345, "error in"=w344) -> ("task out"=w341:refnum<k21>, "error out"=w340:errorcluster)  [unwired: 12 in]
            n147 = call <vilib>:"DAQmx Stop Task.vi"("task/channels in"=w352, "error in"=w338) -> ("task out"=w339:refnum<k21>, "error out"=w337:errorcluster)  [unwired: 12 in]
            n148 = call <vilib>:"DAQmx Clear Task.vi"("task in"=w341, "error in"=w340) -> ("error out"=w351:errorcluster)  [unwired: 13 in]
            n149 = call <vilib>:"DAQmx Clear Task.vi"("task in"=w339, "error in"=w337) -> ("error out"=w349:errorcluster)  [unwired: 13 in]
            n150 = Unbundle By Name(w327) -> ("EventProgressData"=w334:string[][], "CurrentRecordIndicator.CurrentEntry"=w335:string, "StateValue"=w328:T4)
            n151 = control-ref of="Attempt-1"() -> (w332:refnum<vi>)
            n152 = control-ref of="Attempt-2"() -> (w331:refnum<vi>)
            n153 = control-ref of="Attempt-3"() -> (w330:refnum<vi>)
            n154 = control-ref of="Attempt-4"() -> (w329:refnum<vi>)
            n155 = Build Array(w332, w331, w330, w329) -> (w333:refnum<vi>[])
            n156 = call "AccelerationAttemptLEDWinker.vi"("StateValue"=w328, "CurrentEntry"=w335, "EventProgressDataInput"=w334, "inputRefOfLED"=w333) -> ("outputError"=w325:errorcluster)  [unwired: 7 in]
            n157 = Merge Errors "Merge Errors"(w325, w326, w351, w349) -> (w348:errorcluster)
            n158 = local write "Ready"(w350) -> ()
          }
        }
        n159 = Unbundle By Name(w83) -> ("Stop"=w86:bool)
        n160 = in-place {
          in-place-border: w78 -> [w359]
          in-place-border: w86 -> [w358]
          in-place-border: w85 -> [w357]
          n161 = in-place-cluster #12(w83) -> ("StateValue"=w356:T4)
          n162 = Or(x=w358, y=w359) -> (x .or. y?=w360:bool)
          n163 = Select(t=w357, s=w360, f=w356) -> (s? t:f=w361:T4)
          n164 = in-place-cluster #12("StateValue"=w361) -> (w84:T5)
        }
        n165 = Unbundle By Name(w84) -> ("CurrentRecordIndicator"=→"CurrentRecordIndicator":T1, "BestRecordIndicator"=→"BestRecordIndicator":T2)
        n166 = Wait Until Next ms Multiple(millisecond multiple=w92) -> ()  [unwired: 1 out]
      }
    }
    frame #2 {
      n167 = call <vilib>:"Simple Error Handler.vi"("error in (no error)"=w362) -> ()  [unwired: 4 in, 5 out]
    }
  }
